vi "FGV_Initialization.vi"(8 "error in (no error)":errorcluster) -> (0 "error out":errorcluster)   [LabVIEW 2021]
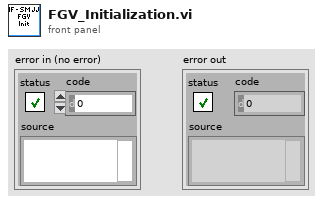
[diagram p1: front panel]
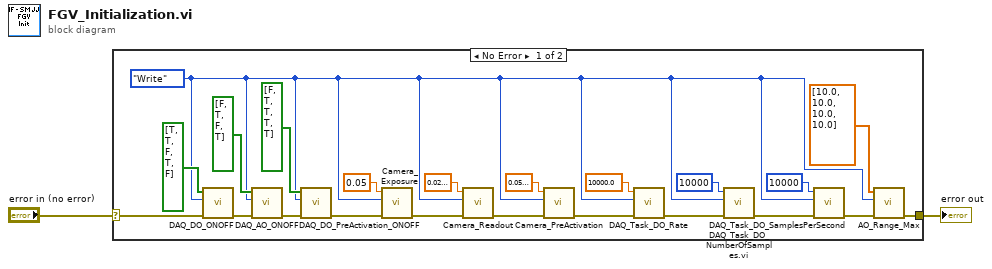
[diagram p0: block diagram]
diagram:
  n1 = case shown="No Error" "error in (no error)" {
    selector: "error in (no error)" -> [w16 w25]
    tunnel: [w3 w25] -> w2
    frame No Error {
      w5 = enum16{"Write", "Read"}."Write" ("Action")
      n2 = call "DAQ_DO_ONOFF.vi"("error in"=w16, "Action"=w5, "DO | ON/OFF"=bool[] [TRUE, TRUE, FALSE, TRUE, FALSE]) -> ("error out"=w8:errorcluster)  [unwired: 7 in, 1 out]
      n3 = call "DAQ_AO_ONOFF.vi"("error in"=w8, "Action"=w5, "AO | ON/OFF"=bool[] [FALSE, TRUE, FALSE, TRUE]) -> ("error out"=w7:errorcluster)  [unwired: 7 in, 1 out]
      n4 = call "DAQ_DO_PreActivation_ONOFF.vi"("error in"=w7, "Action"=w5, "DO | PreActivation ON/OFF"=bool[] [FALSE, TRUE, TRUE, TRUE, TRUE] ("DO | PreActivation")) -> ("error out"=w24:errorcluster)  [unwired: 7 in, 1 out]
      n5 = call "Camera_Exposure.vi"("error in"=w24, "Action"=w5, "Exposure (s)"=0.05 ("Exposure time (s)")) -> ("error out"=w20:errorcluster)  [unwired: 7 in, 1 out]
      n6 = call "Camera_Readout.vi"("error in"=w20, "Action"=w5, "Camera_Readout"=0.020000000000000018 ("Readout time (s)")) -> ("error out"=w22:errorcluster)  [unwired: 7 in, 1 out]
      n7 = call "Camera_PreActivation.vi"("error in"=w22, "Action"=w5, "Camera_PreActivation"=0.050000000000000044 ("Pre-activation time (s)")) -> ("error out"=w14:errorcluster)  [unwired: 7 in, 1 out]
      n8 = call "DAQ_Task_DO_Rate.vi"("error in"=w14, "Action"=w5, "DO_Rate"=10000.0) -> ("error out"=w15:errorcluster)  [unwired: 7 in, 1 out]
      n9 = call "DAQ_Task_DO_NumberOfSamples.vi.vi"("error in"=w15, "Action"=w5, "Samples"=10000) -> ("error out"=w11:errorcluster)  [unwired: 7 in, 1 out]
      n10 = call "DAQ_Task_DO_SamplesPerSecond.vi"("error in"=w11, "Action"=w5, "DO_Task_SamplesPerSec"=u32 10000) -> ("error out"=w6:errorcluster)  [unwired: 7 in, 1 out]
      n11 = call "AO_Range_Max.vi"("error in"=w6, "Action"=w5, "AO | Max"=dbl[] [10.0, 10.0, 10.0, 10.0]) -> ("error out"=w3:errorcluster)  [unwired: 7 in, 1 out]
    }
    frame Error {
    }
  }
  "error out" <- w2
